vi "get_settings_cluster.vi"(8 "error in (no error)":errorcluster, 11 "GenericPlugin in":refnum<class "TrajectoryAN1106117SinglePoint.lvclass">) -> (0 "error out":errorcluster, 2 "settings cluster":variant, 3 "GenericPlugin out":refnum<class "TrajectoryAN1106117SinglePoint.lvclass">)   [LabVIEW 2010, in "TrajectoryAN1106117SinglePoint.lvclass"]
uses:
  TrajectoryAN1106117SinglePoint.lvclass
  TrajectoryAN1106117SinglePoint.lvclass/TrajectoryAN1106117SinglePoint.ctl
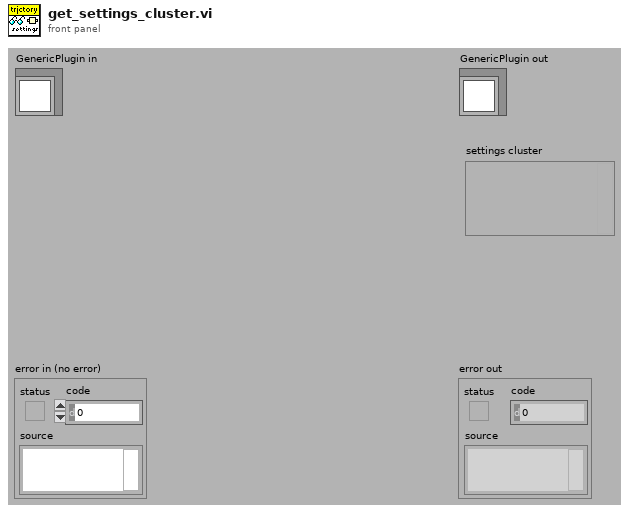
[diagram p1: front panel]
types:
  T1 = typedef "TrajectoryAN1106117SinglePoint.lvclass/settings_cluster.ctl" = cluster{"number of pixels":u32}
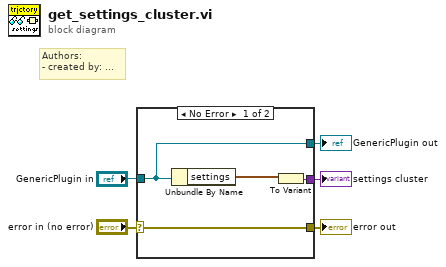
[diagram p0: block diagram]
diagram:
  # "Authors: \n- created by: ..."
  n1 = case shown="No Error" "error in (no error)" {
    selector: "error in (no error)" -> [w7 w11]
    tunnel: [w8 _] -> w5
    tunnel: [w7 w11] -> w3
    tunnel: "GenericPlugin in" -> [w6 w10]
    tunnel: [w6 w10] -> w1
    frame No Error {
      n2 = Unbundle By Name(w6) -> ("settings"=w9:T1)
      n3 = To Variant(anything=w9) -> (Variant=w8:variant)
    }
    frame Error {
    }
  }
  "error out" <- w3
  "GenericPlugin out" <- w1
  "settings cluster" <- w5
